vi "spec_SetGratingByIndex.vi"(8 "error in (no error)":errorcluster, 10 "Grating Index (0 -> n-1)":i32, 11 "LightField Automation in":refnum<class "LightField Automation.lvclass">) -> (0 "error out":errorcluster, 3 "LightField Automation out":refnum<class "LightField Automation.lvclass">)   [LabVIEW 2013, in "LightField Automation.lvclass"]
uses:
  LightField Automation.lvclass
  C:/Program Files/Princeton Instruments/LightField/PrincetonInstruments.LightFieldAddInSupportServices.dll
  Program Files/Princeton Instruments/LightField/PrincetonInstruments.LightFieldAddInSupportServices.dll
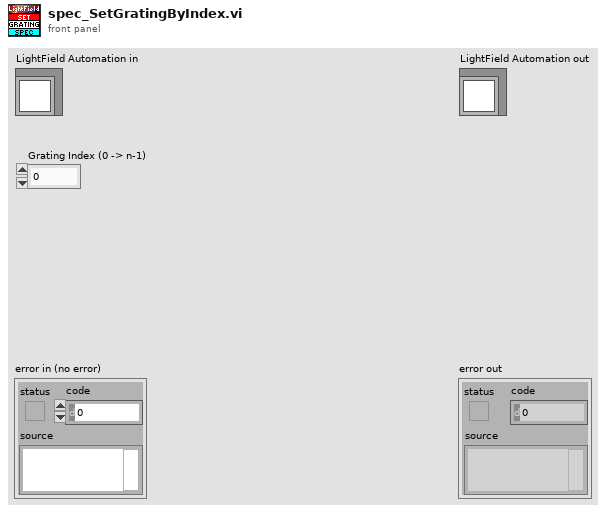
[diagram p1: front panel]
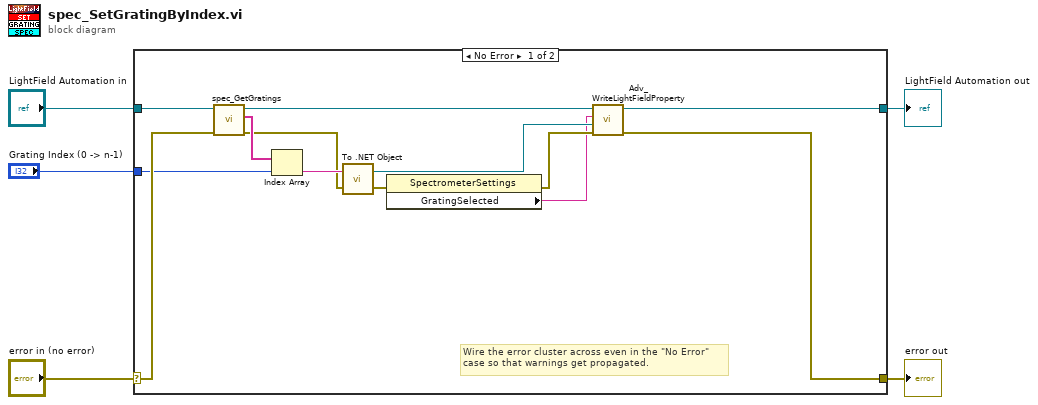
[diagram p0: block diagram]
diagram:
  n1 = case shown="No Error" "error in (no error)" {
    selector: "error in (no error)" -> [w11 w20]
    tunnel: [w14 w20] -> w4
    tunnel: [w13 w19] -> w2
    tunnel: "LightField Automation in" -> [w12 w19]
    tunnel: "Grating Index (0 -> n-1)" -> [w9 _]
    frame No Error {
      # "Wire the error cluster across even in the \"No Error\"\ncase so that warnings get propagated."
      n2 = call "spec_GetGratings.vi"("error in (no error)"=w11, "LightField Automation in"=w12) -> ("error out"=w7:errorcluster, "Gratings"=w10:string[], "LightField Automation out"=w6:refnum<class "LightField Automation.lvclass">)  [unwired: 6 in, 1 out]
      n3 = Index Array(array=w10, index=w9) -> (element=w8:string)
      n4 = call <vilib>:"To .NET Object.vi"("error in (no error)"=w7, "anything"=w8) -> ("error out"=w17:errorcluster, ".NET object"=w18:refnum<k24>)
      n5 = property class="SpectrometerSettings"(error in=w17) -> (error out=w16:errorcluster, "GratingSelected"=w15:string)  [unwired: 1 in, 1 out]
      n6 = call "Adv_WriteLightFieldProperty.vi"("error in (no error)"=w16, "value"=w18, "setting"=w15, "LightField Automation in"=w6) -> ("error out"=w14:errorcluster, "LightField Automation out"=w13:refnum<class "LightField Automation.lvclass">)  [unwired: 6 in]
    }
    frame Error {
    }
  }
  "error out" <- w4
  "LightField Automation out" <- w2
